vi "Mixture.vi"   [LabVIEW 2020]
doc: "Polymorphic VI for mixture models"
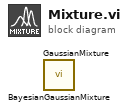
[diagram p0: block diagram]
diagram:
  n1 = call "BayesianGaussianMixture.vi"() -> ()  [unwired: 10 in, 2 out]
  n2 = call "GaussianMixture.vi"() -> ()  [unwired: 10 in, 2 out]
